vi "GUI_resolutionSensitivity.vi"(8 "error in (no error)":errorcluster, 9 "resolution ref":refnum<vi>, 10 "sensitivity ref":refnum<vi>, 11 "Thorlabs_OSA200_64 in":refnum<class "OSA200.lvclass">) -> (0 "error out":errorcluster, 3 "Thorlabs_OSA200_64 out":refnum<class "OSA200.lvclass">)   [LabVIEW 2010, in "OSA200.lvclass"]
uses:
  OSA200.lvclass
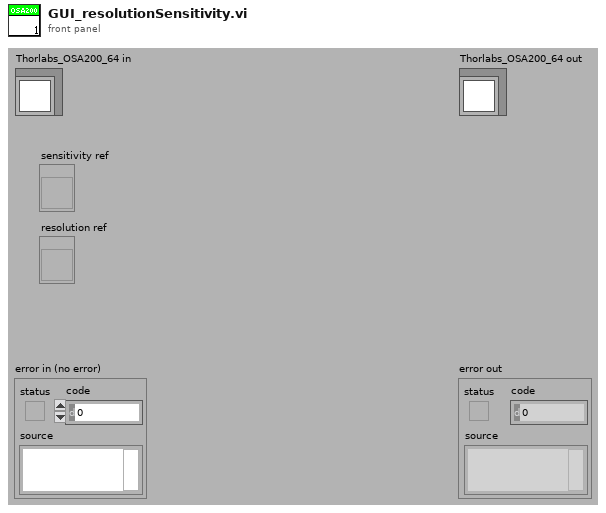
[diagram p1: front panel]
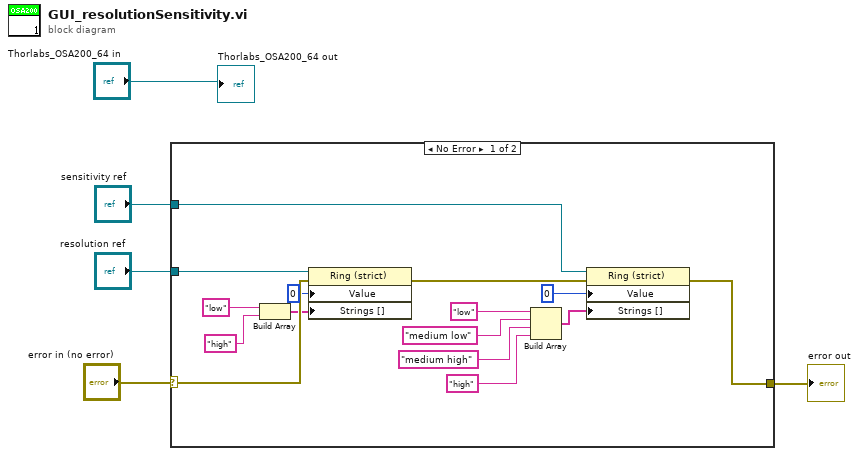
[diagram p0: block diagram]
diagram:
  n1 = case shown="No Error" "error in (no error)" {
    selector: "error in (no error)" -> [w17 w21]
    tunnel: "resolution ref" -> [w20 _]
    tunnel: "sensitivity ref" -> [w16 _]
    tunnel: [w8 w21] -> w2
    frame No Error {
      n2 = Build Array("low", "high") -> (w13:string[])
      n3 = property class="Ring (strict)"(reference=w20, error in=w17, "Value"=u16 0, "Strings []"=w13) -> (error out=w9:errorcluster)  [unwired: 1 out]
      n4 = Build Array("low", "medium low", "medium high" ("element"), "high" ("element")) -> (w12:string[])
      n5 = property class="Ring (strict)"(reference=w16, error in=w9, "Value"=u16 0, "Strings []"=w12) -> (error out=w8:errorcluster)  [unwired: 1 out]
    }
    frame Error {
    }
  }
  "error out" <- w2
  "Thorlabs_OSA200_64 out" <- "Thorlabs_OSA200_64 in"
